vi "AVS_initialise.vi"   [LabVIEW 2018]
uses:
  Global/Global Variables/Data_Display_global.vi
  Instrument_Setup.vi
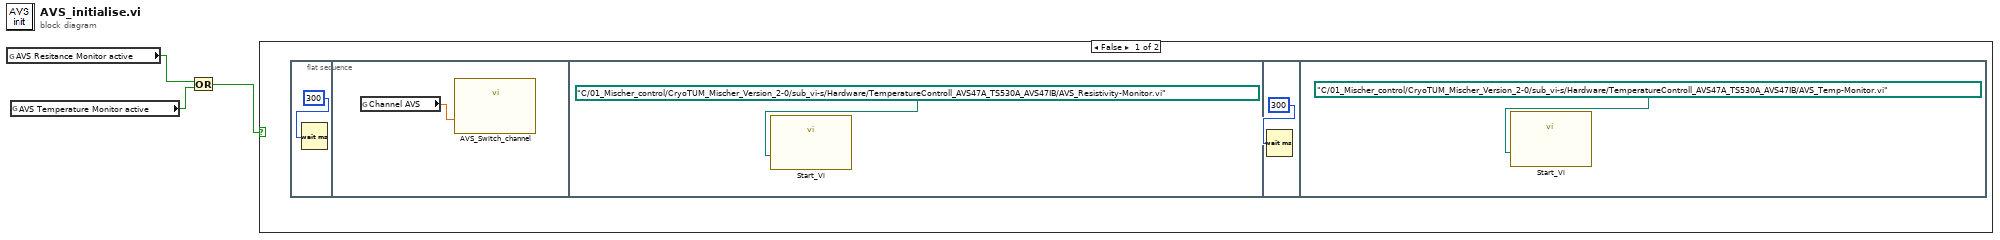
[diagram p0: block diagram]
diagram:
  n1 = global read "Data_Display_global.vi" "AVS Resitance Monitor active"() -> (w3:bool)
  n2 = global read "Data_Display_global.vi" "AVS Temperature Monitor active"() -> (w2:bool)
  n3 = Or(x=w3, y=w2) -> (x .or. y?=w1:bool)
  n4 = case shown="False" w1 {
    frame False {
      n5 = flat-sequence {
        frame #0 {
          n6 = Wait (ms)(milliseconds to wait=300) -> ()  [unwired: 1 out]
        }
        frame #1 {
          n7 = global read "Instrument_Setup.vi" "Channel AVS"() -> (w5:dbl)
          n8 = call "AVS_Switch_channel.vi"("AVS Channel"=w5) -> ()  [unwired: 11 in]
        }
        frame #2 {
          n9 = call "Start_Vi.vi"("VI-Pfad"=path "C:/01_Mischer_control/CryoTUM_Mischer_Version_2-0/sub_vi-s/Hardware/TemperatureControll_AVS47A_TS530A_AVS47IB/AVS_Resistivity-Monitor.vi") -> ()  [unwired: 1 in]
        }
        frame #3 {
          n10 = Wait (ms)(milliseconds to wait=300) -> ()  [unwired: 1 out]
        }
        frame #4 {
          n11 = call "Start_Vi.vi"("VI-Pfad"=path "C:/01_Mischer_control/CryoTUM_Mischer_Version_2-0/sub_vi-s/Hardware/TemperatureControll_AVS47A_TS530A_AVS47IB/AVS_Temp-Monitor.vi") -> ()  [unwired: 1 in]
        }
      }
    }
    frame True {
    }
  }
